vi "weblink handler.vi"(5 "[user-specified font]":T1={"Font Name:"="", "Size"=12, "Strikeout?"=FALSE, "Italic?"=FALSE, "Underline?"=FALSE, "Outline?"=FALSE, "Shadow?"=FALSE, "Bold?"=FALSE}, 6 "Initialize? (f)":bool, 7 "desired font(Application)":T2(ring)=enum."Application Font", 8 "error in (no error)":errorcluster, 9 "Link Color (black)":u32(colorbox), 10 "Link (\"\")":string, 11 "Web\nref":refnum<vi>) -> (0 "error out":errorcluster, 3 "dup Web\nref":refnum<vi>)   [LabVIEW 2011]
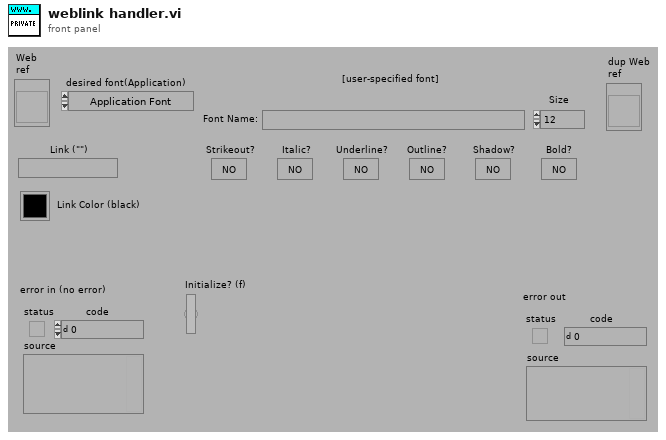
[diagram p1: front panel]
types:
  T1 = cluster{"Font Name:":string, "Size":i16, "Strikeout?":bool, "Italic?":bool, "Underline?":bool, "Outline?":bool, "Shadow?":bool, "Bold?":bool}
  T2 = enum16{"User-specified Font", "Application Font", "System Font", "Dialog Font"}
  T3 = cluster{"left":i16, "top":i16, "right":i16, "bottom":i16}
  T4 = typedef "LVPositionTypeDef.ctl" = cluster{"Left":i32, "Top":i32}
  T5 = typedef "LVBoundsTypeDef.ctl" = cluster{"Width":u32, "Height":u32}
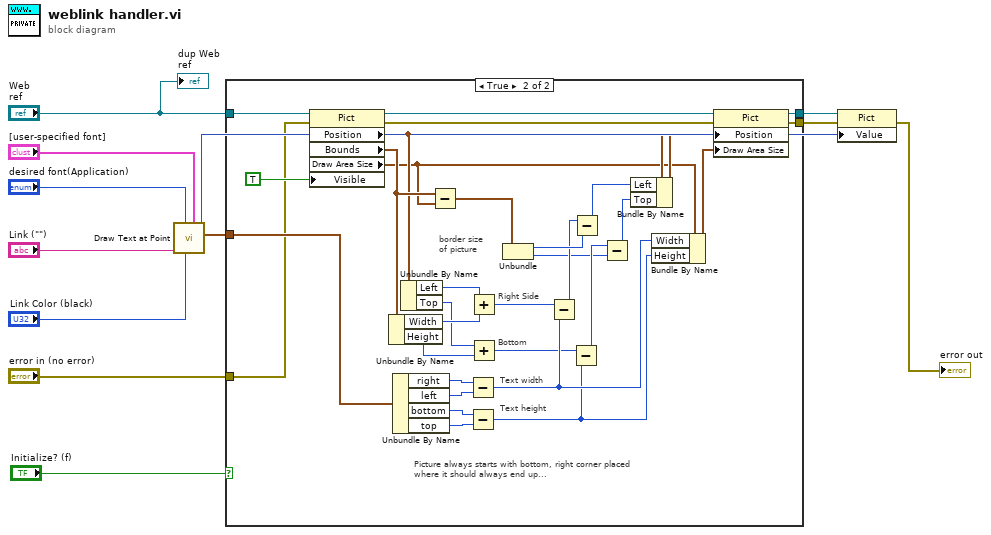
[diagram p0: block diagram]
diagram:
  n1 = call <vilib>:"Draw Text at Point.vi"("[user-specified font]"="[user-specified font]", "text color(black)"="Link Color (black)", "desired font(Application)"="desired font(Application)", "text"="Link (\"\")") -> ("text rect"=w11:T3, "new picture"=w9:picture)  [unwired: 5 in, 1 out]
  n2 = case shown="True" "Initialize? (f)" {
    tunnel: "Web\nref" -> [w14 w46]
    tunnel: w11 -> [_ w40]
    tunnel: [w14 w18] -> w10
    tunnel: "error in (no error)" -> [w13 w17]
    tunnel: [w13 w15] -> w3
    frame False {
    }
    frame True {
      # "border size\nof picture"
      # "Picture always starts with bottom, right corner placed\nwhere it should always end up..."
      # "Text height"
      # "Text width"
      # "Bottom"
      # "Right Side"
      n3 = property on="Property Node" class="Pict"(reference=w46, error in=w17, "Visible"=TRUE) -> (reference out=w45:refnum<vi>, error out=w16:errorcluster, "Position"=w27:T4, "Bounds"=w29:T5, "Draw Area Size"=w26:T5)
      n4 = Unbundle By Name(w29) -> ("Width"=w43:u32, "Height"=w41:u32)
      n5 = Unbundle By Name(w40) -> ("right"=w39:i16, "left"=w38:i16, "bottom"=w37:i16, "top"=w36:i16)
      n6 = Unbundle By Name(w27) -> ("Left"=w44:i32, "Top"=w42:i32)
      n7 = Subtract(x=w29, y=w26) -> (x-y=w25:T5)
      n8 = Subtract(x=w39, y=w38) -> (x-y=w32:i16)
      n9 = Subtract(x=w37, y=w36) -> (x-y=w30:i16)
      n10 = Add(x=w44, y=w43) -> (x+y=w33:u32)
      n11 = Add(x=w42, y=w41) -> (x+y=w31:u32)
      n12 = Unbundle(w25) -> ("Width"=w28:u32, "Height"=w20:u32)
      n13 = Subtract(x=w33, y=w32) -> (x-y=w24:u32)
      n14 = Subtract(x=w31, y=w30) -> (x-y=w21:u32)
      n15 = Subtract(x=w24, y=w28) -> (x-y=w23:u32)
      n16 = Subtract(x=w21, y=w20) -> (x-y=w22:u32)
      n17 = Bundle By Name(cluster=w27, "Left"=w23, "Top"=w22) -> (w35:T4)
      n18 = Bundle By Name(cluster=w26, "Width"=w32, "Height"=w30) -> (w34:T5)
      n19 = property on="Property Node" class="Pict"(reference=w45, error in=w16, "Position"=w35, "Draw Area Size"=w34) -> (reference out=w18:refnum<vi>, error out=w15:errorcluster)
    }
  }
  n20 = property on="Property Node" class="Pict"(reference=w10, error in=w3, "Value"=w9) -> (error out=→"error out":errorcluster)  [unwired: 1 out]
  "dup Web\nref" <- "Web\nref"
